vi "_builtins_arrange_node.vi"(8 "error in (no error)":errorcluster, 10 "Arrange":T1, 11 "Node in":refnum<vi>) -> (0 "error out":errorcluster, 3 "Node out":refnum<vi>)   [LabVIEW 2019, in "Script.lvlib"]
doc: "Arrange node terminal positions and adjust for custom terminal offsets.\n\nCreated by: Ryan Pacini"
uses:
  Script.lvlib
  _builtins_arrange.ctl
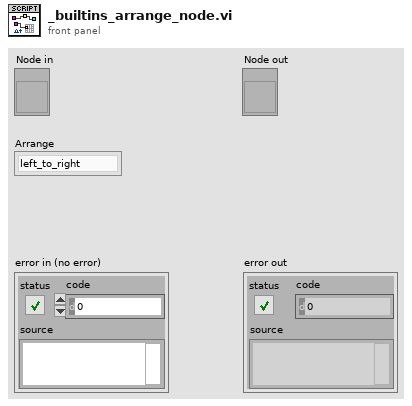
[diagram p1: front panel]
types:
  T1 = typedef "Script.lvlib/_builtins_arrange.ctl" = enum8{"left_to_right", "right_to_left"}
  T2 = cluster{"Position":cluster{"h":i16, "v":i16}, "Flags":i32, "Type":enum32{"LooseEnd", "Endpoint", "Bend", "Junction"}, "Up Joint Index":i16, "Down Joint Index":i16, "Left Joint Index":i16, "Right Joint Index":i16}[]
  T3 = typedef "LVRectTypeDef.ctl" = cluster{"Left":i16, "Top":i16, "Right":i16, "Bottom":i16}
  T4 = typedef "LVPositionTypeDef.ctl" = cluster{"Left":i32, "Top":i32}
  T5 = cluster{"Left":i32, "Top":i32, "Right":i32, "Bottom":i32}
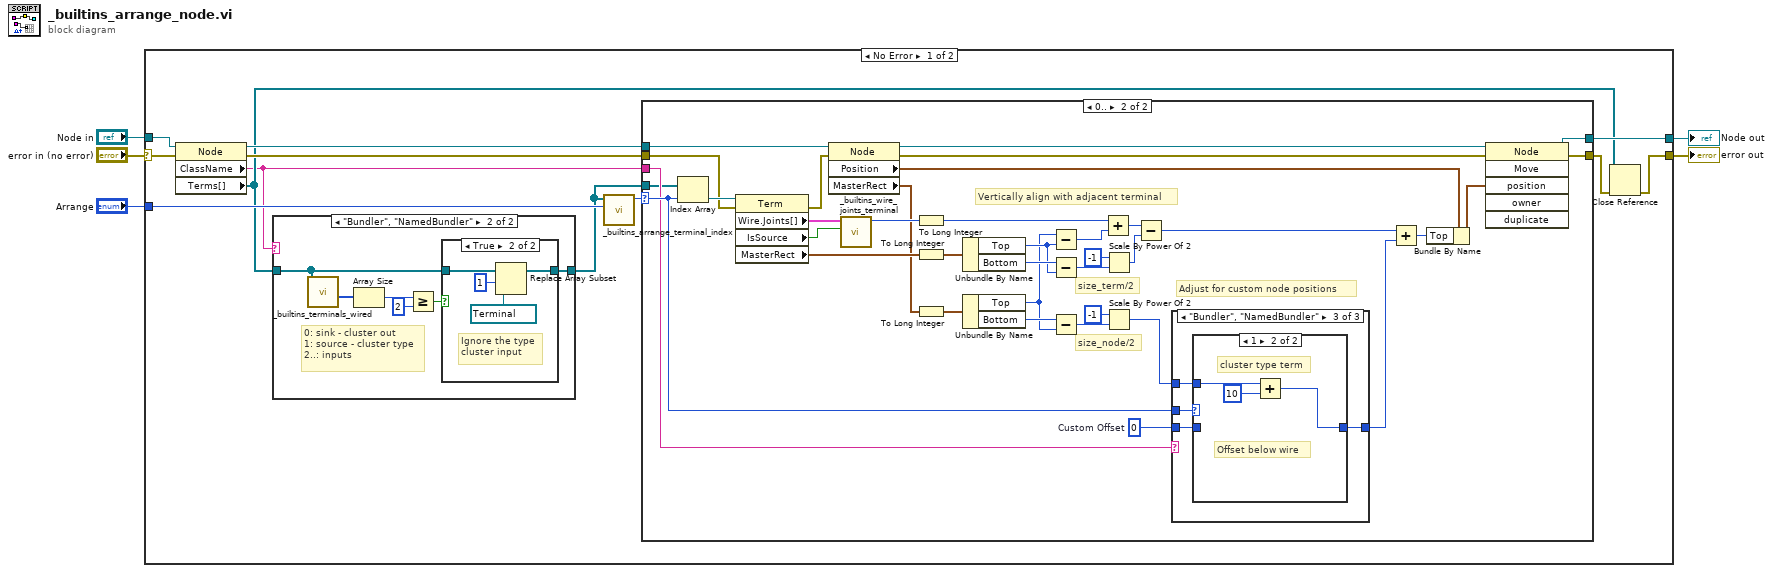
[diagram p0: block diagram]
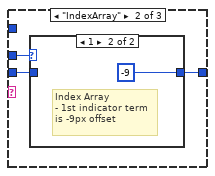
[diagram p6: hidden frame]
diagram:
  n1 = case shown="No Error" "error in (no error)" {
    selector: "error in (no error)" -> [w12 w83]
    tunnel: "Arrange" -> [w13 _]
    tunnel: "Node in" -> [w11 w84]
    tunnel: [w10 w83] -> w2
    tunnel: [w9 w84] -> w1
    frame No Error {
      n2 = property class="Node"(reference=w11, error in=w12) -> (reference out=w17:refnum<vi>, error out=w16:errorcluster, "ClassName"=w6:string, "Terms[]"=w8:refnum<vi>[])
      n3 = case shown="\"Bundler\", \"NamedBundler\"" w6 {
        tunnel: w8 -> [w18 w23]
        tunnel: [w18 w24] -> w7
        frame Default {
        }
        frame "Bundler", "NamedBundler" {
          # "0: sink - cluster out\n1: source - cluster type\n2..: inputs"
          n4 = call "_builtins_terminals_wired.vi"("Terminals"=w23) -> ("Node Input indexes"=w21:i32[])  [unwired: 8 in, 2 out]
          n5 = Array Size(array=w21) -> (size(s)=w19:i32)
          n6 = Greater Or Equal?(x=w19, y=2) -> (x >= y?=w20:bool)
          n7 = case shown="True" w20 {
            tunnel: [w25 w29] -> w24
            tunnel: w23 -> [w25 w28]
            frame False {
            }
            frame True {
              # "Ignore the type\ncluster input"
              n8 = Replace Array Subset(array=w28, new element=refnum<vi> refnum ("new element/subarray"), index=1) -> (w29:refnum<vi>[])
            }
          }
        }
      }
      n9 = call "_builtins_arrange_terminal_index.vi"("Arrange"=w13, "Terminals"=w7) -> ("Terminal Index"=w15:i32)  [unwired: 9 in]
      n10 = case shown="0.." w15 {
        selector: w15 -> [_ w46]
        tunnel: [w31 w68] -> w14
        tunnel: w17 -> [w30 w63]
        tunnel: w16 -> [w31 w58]
        tunnel: w7 -> [_ w42]
        tunnel: w6 -> [_ w45]
        tunnel: [w30 w43] -> w9
        frame ..-1 {
        }
        frame 0.. {
          w48 = 0  # Custom Offset
          # "Adjust for custom node positions"
          # "size_node/2"
          # "size_term/2"
          # "Vertically align with adjacent terminal"
          n11 = Index Array(array=w42, index=w46) -> (element=w60:refnum<vi>)
          n12 = property class="Term"(reference=w60, error in=w58) -> (error out=w59:errorcluster, "Wire.Joints[]"=w61:T2, "IsSource"=w44:bool, "MasterRect"=w57:T3)  [unwired: 1 out]
          n13 = property class="Node"(reference=w63, error in=w59) -> (reference out=w66:refnum<vi>, error out=w67:errorcluster, "Position"=w65:T4, "MasterRect"=w41:T3)
          n14 = call "_builtins_wire_joints_terminal.vi"("Is Source?"=w44, "Joints"=w61) -> ("Vertical Position"=w62:i16)  [unwired: 8 in, 1 out]
          n15 = To Long Integer(number=w62) -> (32bit integer=w55:i32)
          n16 = To Long Integer(number=w57) -> (32bit integer=w53:T5)
          n17 = To Long Integer(number=w41) -> (32bit integer=w39:T5)
          n18 = Unbundle By Name(w53) -> ("Top"=w52:i32, "Bottom"=w56:i32)
          n19 = Unbundle By Name(w39) -> ("Top"=w38:i32, "Bottom"=w40:i32)
          n20 = Subtract(x=w38, y=w52) -> (x-y=w54:i32)
          n21 = Subtract(x=w56, y=w52) -> (x-y=w34:i32)
          n22 = Subtract(x=w40, y=w38) -> (x-y=w37:i32)
          n23 = Add(x=w55, y=w54) -> (x+y=w51:i32)
          n24 = Scale By Power Of 2(n=i16 -1, x=w34) -> (x*2^n=w33:i32)
          n25 = Scale By Power Of 2(n=i16 -1, x=w37) -> (x*2^n=w32:i32)
          n26 = Subtract(x=w51, y=w33) -> (x-y=w50:i32)
          n27 = case shown="\"Bundler\", \"NamedBundler\"" w45 {
            tunnel: w46 -> [_ w72 w78]
            tunnel: [w69 w71 w77] -> w47
            tunnel: w48 -> [w69 w70 w76]
            tunnel: w32 -> [_ _ w75]
            frame Default {
            }
            frame "IndexArray" {
              n28 = case shown="1" w72 {
                tunnel: [w73 -9 ("Vertical Offset")] -> w71
                tunnel: w70 -> [w73 _]
                frame Default {
                }
                frame 1 {
                  # "Index Array\n- 1st indicator term\nis -9px offset"
                }
              }
            }
            frame "Bundler", "NamedBundler" {
              n29 = case shown="1" w78 {
                tunnel: [w79 w80] -> w77
                tunnel: w76 -> [w79 _]
                tunnel: w75 -> [_ w82]
                frame Default {
                }
                frame 1 {
                  # "cluster type term"
                  # "Offset below wire"
                  n30 = Add(x=w82, y=10 ("Vertical Offset")) -> (x+y=w80:i32)
                }
              }
            }
          }
          n31 = Add(x=w50, y=w47) -> (x+y=w49:i32)
          n32 = Bundle By Name(cluster=w65, "Top"=w49) -> (w64:T4)
          n33 = invoke class="Node" method="Move"(reference=w66, error in=w67, "position"=w64) -> (reference out=w43:refnum<vi>, error out=w68:errorcluster)  [unwired: 3 in, 4 out]
        }
      }
      n34 = Close Reference(reference=w8, error in (no error)=w14) -> (error out=w10:errorcluster)
    }
    frame Error {
    }
  }
  "error out" <- w2
  "Node out" <- w1
